vi "single-point-fft.vi"() -> ()   [LabVIEW 2024]
doc: "This example demonstrates how to acquire a single buffer of voltage measurements using a DAQmx device.\n\nFor instructions on how to connect your signals to the DAQ device, refer to your device documentation."
uses:
  <vilib>/Utility/error.llb/DialogType.ctl
  <vilib>/DAQmx/read.llb/DAQmx Read (Analog Wfm 1Chan NSamp).vi
  <vilib>/DAQmx/create/channels.llb/DAQmx Create Channel (AI-Voltage-Basic).vi
  <vilib>/DAQmx/configure/timing.llb/DAQmx Timing (Sample Clock).vi
  <vilib>/DAQmx/configure/task.llb/DAQmx Configure Logging (TDMS).vi
  <vilib>/DAQmx/configure/trigger.llb/DAQmx Start Trigger (Digital Edge).vi
  <vilib>/DAQmx/configure/trigger.llb/DAQmx Start Trigger (Time).vi
  <vilib>/DAQmx/configure/trigger.llb/DAQmx Start Trigger (Analog Edge).vi
  <vilib>/DAQmx/configure/trigger.llb/DAQmx Reference Trigger (Digital Edge).vi
  <vilib>/DAQmx/configure/trigger.llb/DAQmx Reference Trigger (Analog Edge).vi
  <vilib>/DAQmx/miscellaneous.llb/DAQmx Fill In Error Info.vi
  <vilib>/express/express analysis/Spectral/Block/exnSpectralBlock spectral measurements power poly.vi
  <vilib>/express/express analysis/Spectral/Block/exnSpectralBlock spectral measurements power WFM.vi
  <vilib>/express/express analysis/Spectral/XNode/ExpressSpectralMeasurementsBlockNode.xnode
  <resource>/objmgr/daqmx.rc
panel:
  out "velocity dt":waveform(dbl)(graph)
  out "FFT Graph":cluster{"f0":dbl, "df":dbl, "magnitude":dbl[]}(graph)
  out "Y":dbl[](array[numeric])
  out "dt":dbl
  out "t0":timestamp
  in  "Trigger Type":T1(tab)
  in  "Digital Start Trigger Edge":i32(ring)=10280 caption="Edge" items=["Rising"=10280, "Falling"=10171]
  in  "Digital Start Trigger Source":tag="/Dev1/PFI0" caption="Source"
  in  "Digital Pause Trigger Pause When":i32(ring)=10192 caption="Pause When" items=["High"=10192, "Low"=10214]
  in  "Digital Pause Trigger Source":tag="/Dev1/PFI0" caption="Source"
  in  "Digital Reference Trigger Source":tag="/Dev1/PFI0" caption="Source"
  in  "Digital Reference Trigger Edge":i32(ring)=10280 caption="Edge" items=["Rising"=10280, "Falling"=10171]
  in  "Digital Reference Pretrigger Samples":u32 caption="Pretrigger Samples"
  in  "Analog Start Trigger Level":dbl caption="Level" format="%0.2f"
  in  "Analog Start Trigger Hysteresis":dbl caption="Hysteresis" format="%.2f"
  in  "Analog Start Trigger Slope":i32(ring)=10280 caption="Slope" items=["Rising"=10280, "Falling"=10171]
  in  "Analog Start Trigger Source":string="APFI0" caption="Source"
  in  "Analog Pause Trigger Source":string="APFI0" caption="Source"
  in  "Analog Pause Trigger Pause When":i32(ring)=10093 caption="Pause When" items=["Above Level"=10093, "Below Level"=10107]
  in  "Analog Pause Trigger Level":dbl caption="Level" format="%.2f"
  in  "Analog Reference Trigger Source":string="APFI0" caption="Source"
  in  "Analog Reference Trigger Level":dbl caption="Level" format="%.2f"
  in  "Analog Reference Trigger Slope":i32(ring)=10280 caption="Slope" items=["Rising"=10280, "Falling"=10171]
  in  "Analog Reference Pretrigger Samples":u32 caption="Pretrigger Samples"
  in  "When":timestamp
  in  "Select Time\nManually":bool
  in  "TDMS File Path":path
  in  "Number of Samples":i32=100
  in  "Sample Rate":dbl=1000.0
  in  "Sample Clock Source":tag="OnboardClock"
  in  "Terminal Configuration":i32(ring)=-1 items=["default"=-1, "RSE"=10083, "NRSE"=10078, "Differential"=10106, "Pseudodifferential"=12529]
  in  "Max Voltage":dbl=5.0
  in  "Min Voltage":dbl=-5.0
  in  "Physical Channel":tag="Dev1/ai0"
  out "Actual Sample Rate":dbl=1000.0 format="%0.2f"
  in  "Logging Mode":i32(ring)=10231 items=["Off"=10231, "Log and Read"=15842]
  # "Channel Settings"
  # "Acquired Data"
  # "Timing Settings"
  # "Trigger Settings"
  # "Logging Settings"
  # "To enable triggers, select a tab above, and configure the settings.\n\nNot all hardware supports all trigger types. Refer to your device documentation for more information."
  # "If time is not manually set, task will begin after 10 seconds"
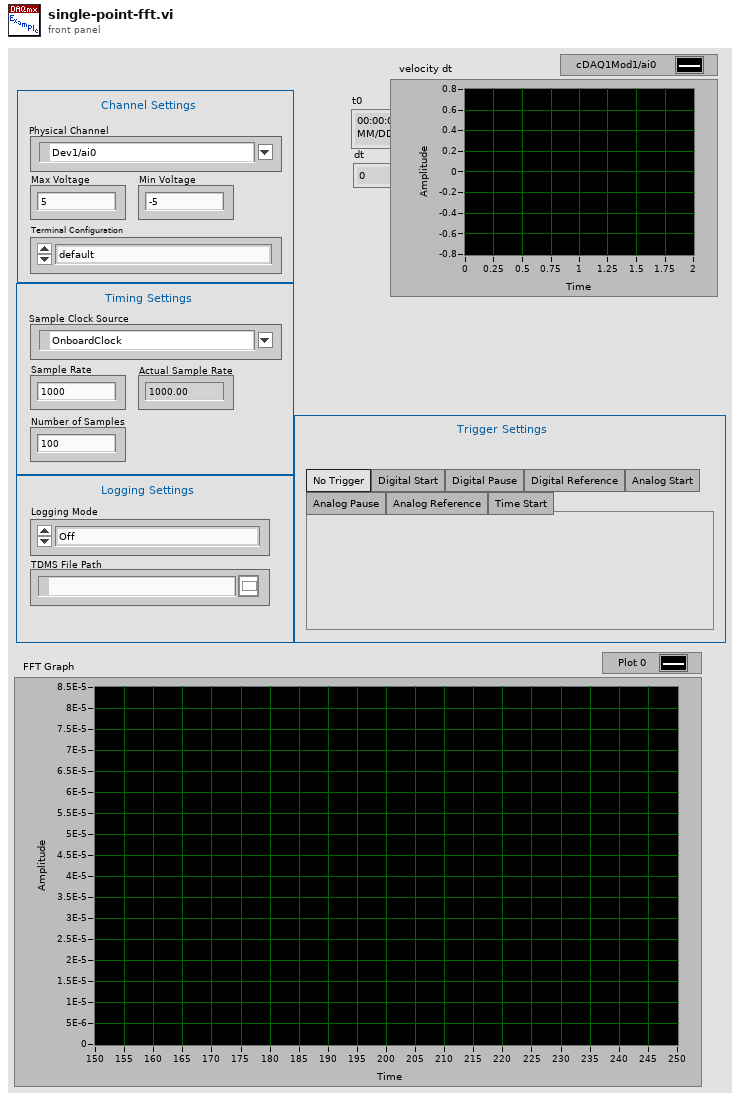
[diagram p1: front panel]
types:
  T1 = enum32{"No Trigger", "Digital Start", "Digital Pause", "Digital Reference", "Analog Start", "Analog Pause", "Analog Reference", "Time Start"}
  T2 = typedef "DialogType.ctl" = u16
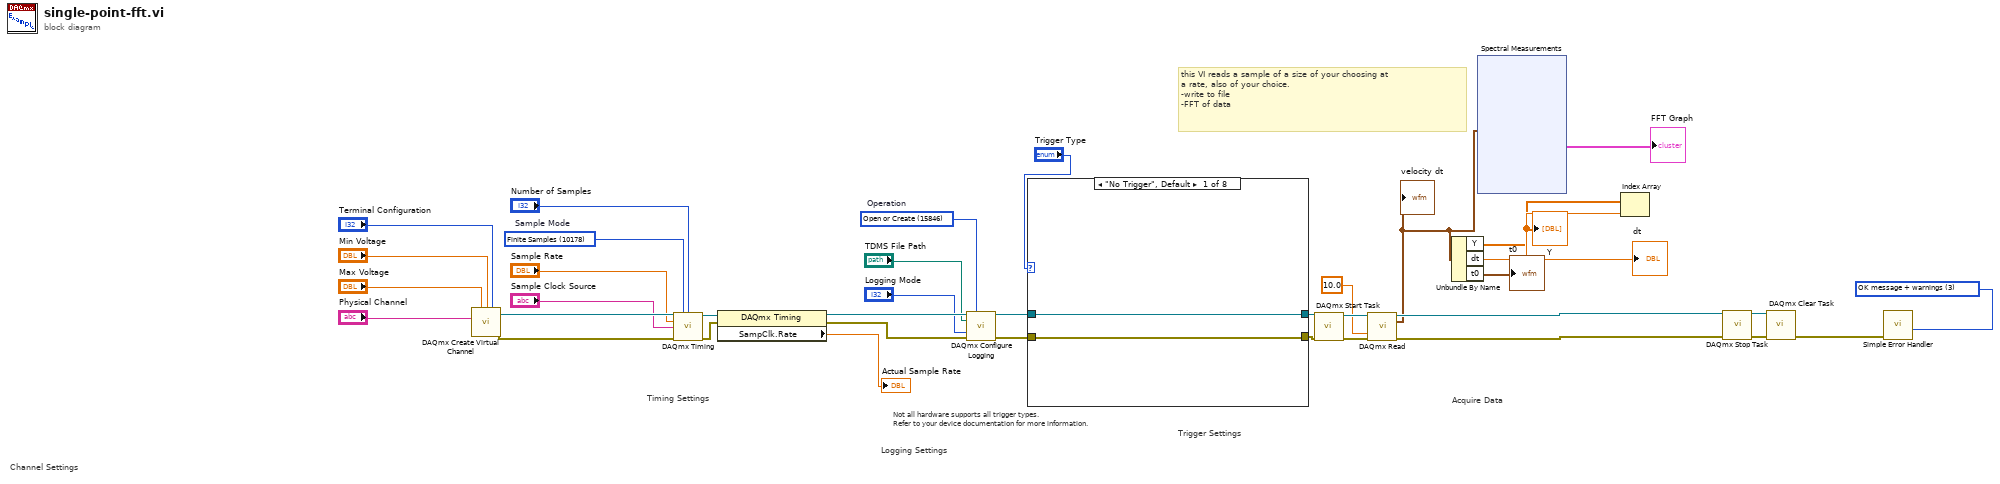
[diagram p0: block diagram]
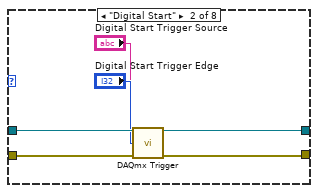
[diagram p2: hidden frame]
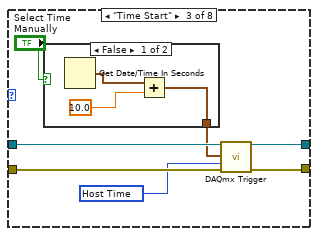
[diagram p3: hidden frame]
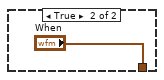
[diagram p4: hidden frame]
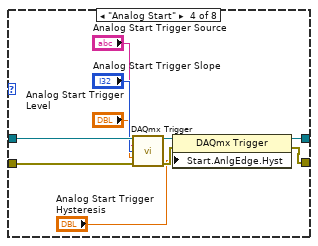
[diagram p5: hidden frame]
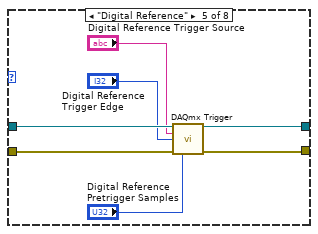
[diagram p6: hidden frame]
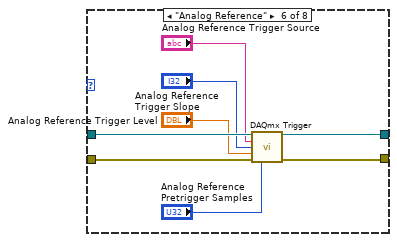
[diagram p7: hidden frame]
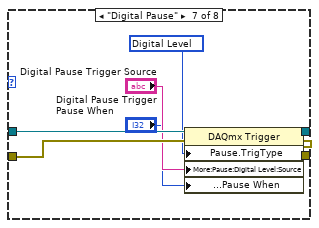
[diagram p8: hidden frame]
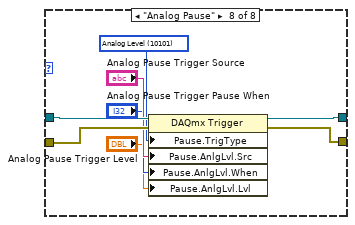
[diagram p9: hidden frame]
diagram:
  w12 = T2 3 items=["no dialog", "OK message", "continue or stop message", "OK message + warnings", "continue/stop + warnings"] ("type of dialog (OK msg:1)")
  w30 = 15846 items=["Open"=10437, "Open or Create"=15846, "Create or Replace"=15847, "Create"=15848]  # Operation
  w35 = 10178 items=["Finite Samples"=10178, "Continuous Samples"=10123, "Hardware Timed Single Point"=12522]  # Sample Mode
  # "this VI reads a sample of a size of your choosing at \na rate, also of your choice.\n-write to file\n-FFT of data"
  # "Not all hardware supports all trigger types.\nRefer to your device documentation for more information."
  # "Trigger Settings"
  # "Acquire Data"
  # "Timing Settings"
  # "Channel Settings"
  # "Logging Settings"
  n1 = call-poly <vilib>:"DAQmx Create Virtual Channel.vi"("maximum value"="Max Voltage", "minimum value"="Min Voltage", "input terminal configuration"="Terminal Configuration", "physical channels"="Physical Channel") -> ("task out"=w33:refnum<k21>, "error out"=w34:errorcluster)  [unwired: 10 in]
  n2 = call-poly <vilib>:"DAQmx Timing.vi"("task/channels in"=w33, "sample mode"=w35, "samples per channel"="Number of Samples", "rate"="Sample Rate", "source"="Sample Clock Source", "error in"=w34) -> ("task out"=w37:refnum<k21>, "error out"=w36:errorcluster)  [unwired: 8 in]
  n3 = property on="Property Node" class="DAQmx Timing"(reference=w37, error in=w36) -> (reference out=w32:refnum<k21>, error out=w31:errorcluster, "SampClk.Rate"=→"Actual Sample Rate":dbl)
  n4 = call-poly <vilib>:"DAQmx Configure Logging.vi"("task/channels in"=w32, "operation"=w30, "file path"="TDMS File Path", "logging mode"="Logging Mode", "error in"=w31) -> ("task out"=w10:refnum<k21>, "error out"=w9:errorcluster)  [unwired: 9 in]
  n5 = case shown="\"No Trigger\", Default" "Trigger Type" {
    tunnel: w10 -> [w39 w45 w52 w66 w73 w81 w88 w96]
    tunnel: w9 -> [w38 w44 w51 w65 w72 w80 w85 w93]
    tunnel: [w39 w43 w50 w63 w71 w79 w87 w95] -> w8
    tunnel: [w38 w42 w49 w62 w70 w78 w86 w94] -> w7
    frame "No Trigger", Default {
    }
    frame "Digital Start" {
      n6 = call-poly <vilib>:"DAQmx Trigger.vi"("task/channels in"=w45, "source"="Digital Start Trigger Source", "edge"="Digital Start Trigger Edge", "error in"=w44) -> ("task out"=w43:refnum<k21>, "error out"=w42:errorcluster)  [unwired: 10 in]
    }
    frame "Time Start" {
      w48 = 16126 items=["Host Time"=16126, "I/O Device Time"=16127] ("timescale")
      n7 = case shown="False" "Select Time\nManually" {
        tunnel: [w54 "When"] -> w46
        frame False {
          n8 = Get Date/Time In Seconds() -> (seconds since 1Jan1904=w55:timestamp)
          n9 = Add(x=w55, y=10.0) -> (x+y=w54:timestamp)
        }
        frame True {
        }
      }
      n10 = call-poly <vilib>:"DAQmx Trigger.vi"("task/channels in"=w52, "when"=w46, "timescale"=w48, "error in"=w51) -> ("task out"=w50:refnum<k21>, "error out"=w49:errorcluster)  [unwired: 10 in]
    }
    frame "Analog Start" {
      n11 = call-poly <vilib>:"DAQmx Trigger.vi"("task/channels in"=w66, "source"="Analog Start Trigger Source", "slope"="Analog Start Trigger Slope", "level"="Analog Start Trigger Level", "error in"=w65) -> ("task out"=w61:refnum<k21>, "error out"=w60:errorcluster)  [unwired: 9 in]
      n12 = property class="DAQmx Trigger"(reference=w61, error in=w60, "Start.AnlgEdge.Hyst"="Analog Start Trigger Hysteresis") -> (reference out=w63:refnum<k21>, error out=w62:errorcluster)
    }
    frame "Digital Reference" {
      n13 = call-poly <vilib>:"DAQmx Trigger.vi"("task/channels in"=w73, "source"="Digital Reference Trigger Source", "edge"="Digital Reference Trigger Edge", "error in"=w72, "pretrigger samples per channel"="Digital Reference Pretrigger Samples") -> ("task out"=w71:refnum<k21>, "error out"=w70:errorcluster)  [unwired: 9 in]
    }
    frame "Analog Reference" {
      n14 = call-poly <vilib>:"DAQmx Trigger.vi"("task/channels in"=w81, "source"="Analog Reference Trigger Source", "slope"="Analog Reference Trigger Slope", "level"="Analog Reference Trigger Level", "error in"=w80, "pretrigger samples per channel"="Analog Reference Pretrigger Samples") -> ("task out"=w79:refnum<k21>, "error out"=w78:errorcluster)  [unwired: 8 in]
    }
    frame "Digital Pause" {
      w84 = 10152 items=["Analog Level"=10101, "Analog Window"=10103, "Digital Level"=10152, "Digital Pattern"=10398, "None"=10230] ("Pause.TrigType")
      n15 = property class="DAQmx Trigger"(reference=w88, error in=w85, "Pause.TrigType"=w84, "More:Pause:Digital Level:Source"="Digital Pause Trigger Source", "More:Pause:Digital Level:Pause When"="Digital Pause Trigger Pause When") -> (reference out=w87:refnum<k21>, error out=w86:errorcluster)
    }
    frame "Analog Pause" {
      w92 = 10101 items=["Analog Level"=10101, "Analog Window"=10103, "Digital Level"=10152, "Digital Pattern"=10398, "None"=10230] ("Pause.TrigType")
      n16 = property class="DAQmx Trigger"(reference=w96, error in=w93, "Pause.TrigType"=w92, "Pause.AnlgLvl.Src"="Analog Pause Trigger Source", "Pause.AnlgLvl.When"="Analog Pause Trigger Pause When", "Pause.AnlgLvl.Lvl"="Analog Pause Trigger Level") -> (reference out=w95:refnum<k21>, error out=w94:errorcluster)
    }
  }
  n17 = call <vilib>:"DAQmx Start Task.vi"("task/channels in"=w8, "error in"=w7) -> ("task out"=w29:refnum<k21>, "error out"=w28:errorcluster)  [unwired: 12 in]
  n18 = call-poly <vilib>:"DAQmx Read.vi"("task/channels in"=w29, "timeout"=10.0, "error in"=w28) -> ("task out"=w14:refnum<k21>, "data"=w1:waveform(dbl), "error out"=w13:errorcluster)  [unwired: 10 in]
  "velocity dt" <- w1
  n19 = Unbundle By Name(w1) -> ("Y"=w3:dbl[], "dt"=w4:dbl, "t0"=→"t0":timestamp)
  "dt" <- w4
  "Y" <- w3
  n20 = xnode "Spectral Measurements"("Signals"=w1) -> ("Power Spectrum"=→"FFT Graph":cluster{"f0":dbl, "df":dbl, "magnitude":dbl[]})  [unwired: 2 in, 2 out]
  n21 = Index Array(array=w3, index=w4) -> ()  [unwired: 1 out]
  n22 = call <vilib>:"DAQmx Stop Task.vi"("task/channels in"=w14, "error in"=w13) -> ("task out"=w16:refnum<k21>, "error out"=w15:errorcluster)  [unwired: 12 in]
  n23 = call <vilib>:"DAQmx Clear Task.vi"("task in"=w16, "error in"=w15) -> ("error out"=w27:errorcluster)  [unwired: 13 in]
  n24 = call <vilib>:"Simple Error Handler.vi"("type of dialog (OK msg:1)"=w12, "error in (no error)"=w27) -> ()  [unwired: 3 in, 5 out]
